vi "Desktop Main.vi"() -> ()   [LabVIEW 2019]
doc: "Sends commands and instructions through UDP communication to the myRIO in order to move the motors"
panel:
  out "Tab of colors":i32[][](array[numeric])
  out "Camera 4":T1(plugin-control)
  out "Camera 3":T1(plugin-control)
  out "Camera 2":T1(plugin-control)
  out "Camera 1":T1(plugin-control)
  in  "RESET":bool
  out "Random":string[](array[string])
  out "Commands to Execute":string[](array[string])
  out "Time to execute \n(in second)":dbl(slide) scale=0.014..14.0
  in  "Speed":string(combo)="Slow"
  in  "Difficulty for random":string(combo)="Easy"
  in  "Unrandomize":bool
  in  "Random":bool
  in  "Touche U'":bool
  in  "Touche U":bool
  in  "Touche D'":bool
  in  "Touche D":bool
  in  "Touche L'":bool
  in  "Touche L":bool
  in  "Touche B'":bool
  in  "Touche B":bool
  in  "Touche R'":bool
  in  "Touche F'":bool
  in  "Touche R":bool
  in  "Solve":bool
  in  "Touche F":bool
  in  "Tab cmd forcées":string[](array[string])
  in  "GO Tableau forcé":bool
  in  "Stop Button":bool
  out "error out":errorcluster
  in  "Target IP Address":string="172.22.11.2"
  # "Overview: Resolve a Rubik's cube or send some commands using User Datagram Protocol (UDP). The data of this \"Desktop Main\" is sent to the myRIO target.\n\nInstructions:\n1. Ensure RT Main.vi is already running.\n2. Run this VI.\n3. Click on the function you want.\n4. Observe the Rubik's cube moving.\n5. Click Stop to stop both VIs."
  # "Move a face"
  # "Difficulty for randomize"
  # "Easy : 5 moves\nMedium : 15 moves\nHard : 25 moves\nHardcore : 50 moves"
  # "List of commands to execute"
  # "1. Write in the tab the commands you want to execute\n    (F, F', L, L', R, R', B, B', U, U', D, D')\n\n2. Click on \"LAUNCH\"\n\n3. Click on \"RESET COMMANDS\" to reset the keys you entered"
  # "s"
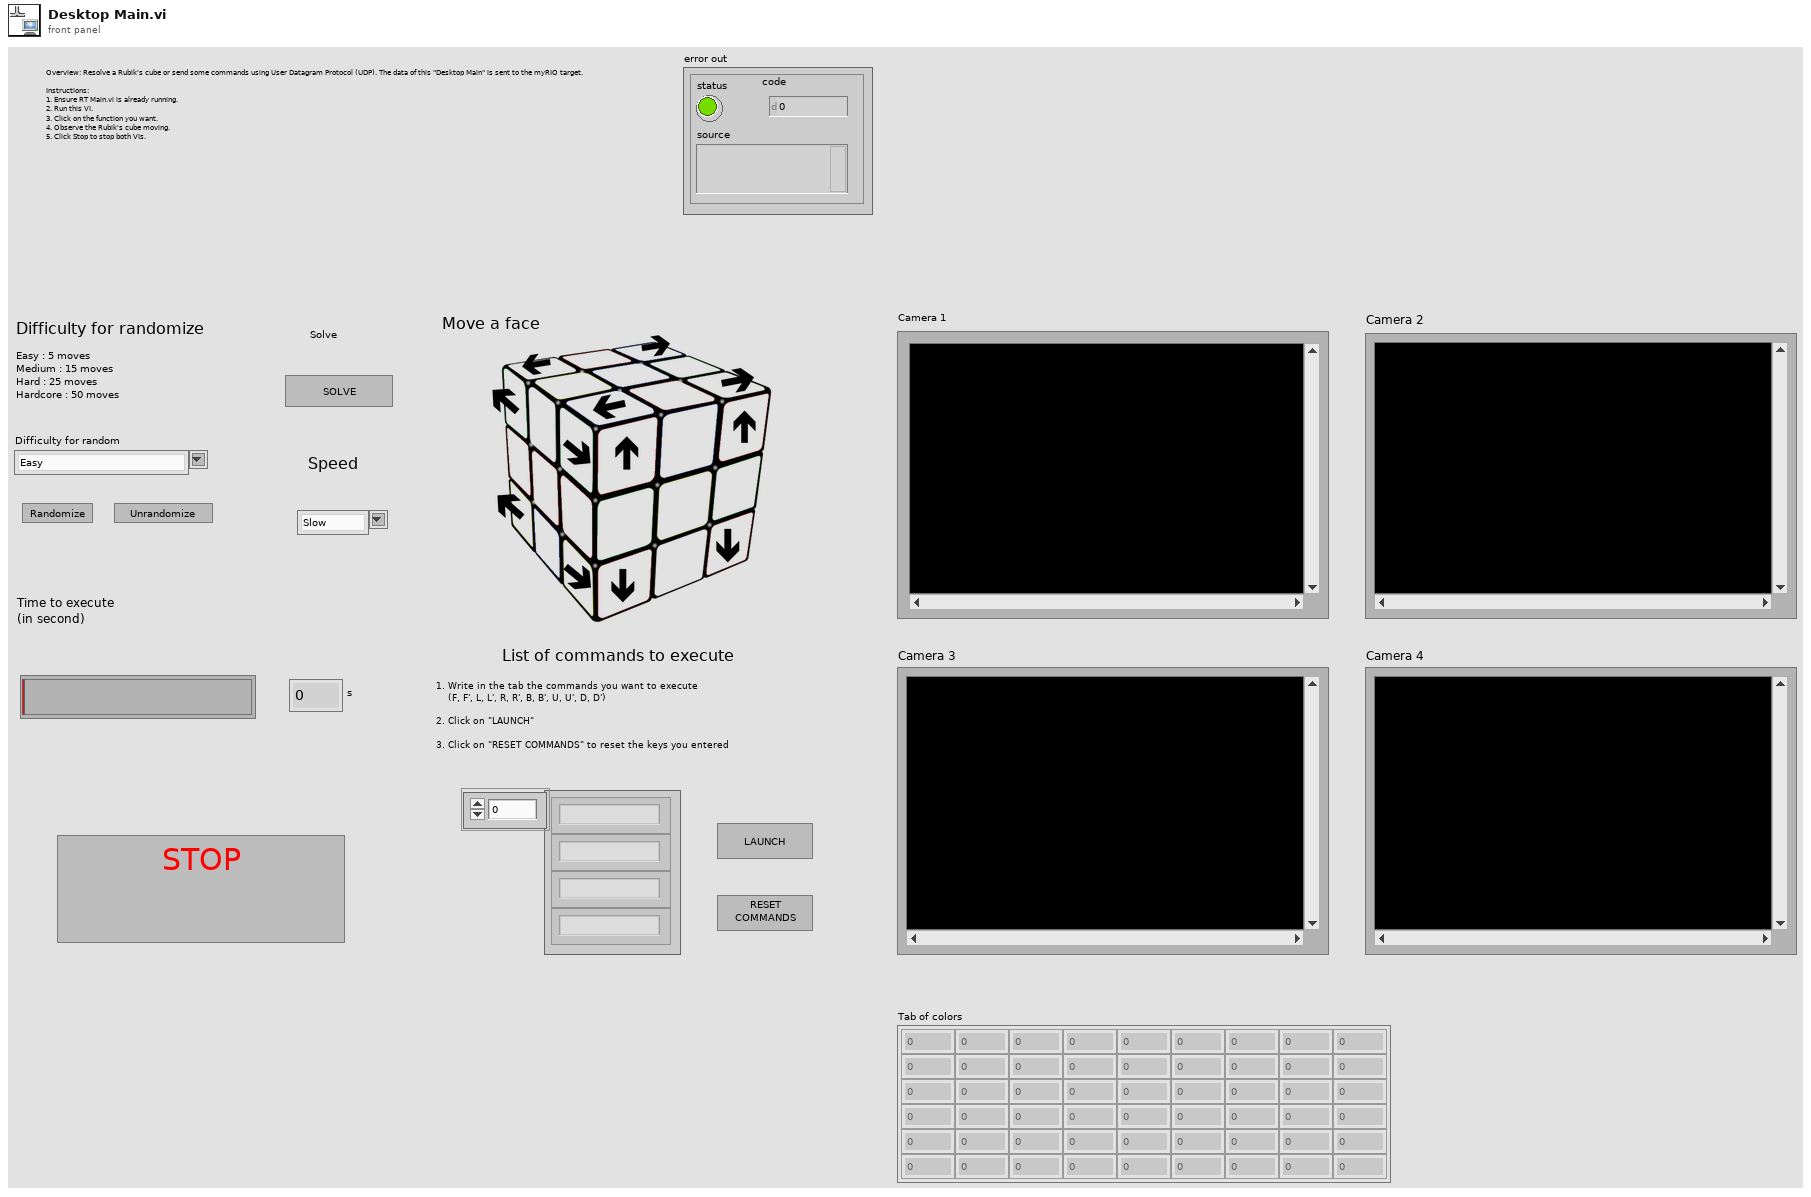
[diagram p1: front panel]
types:
  T1 = typedef "IMAQ Image.ctl" = refnum<image>
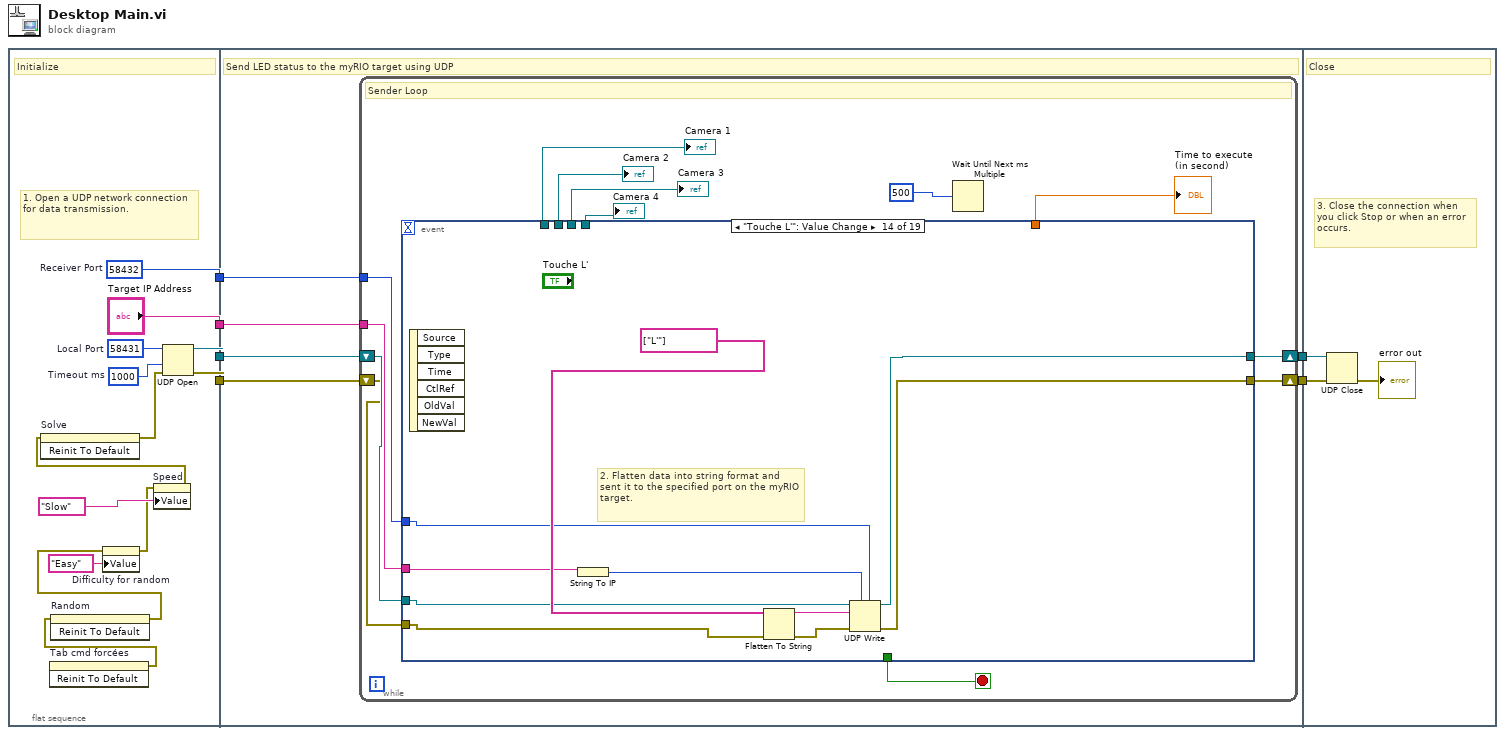
[diagram p0: block diagram]
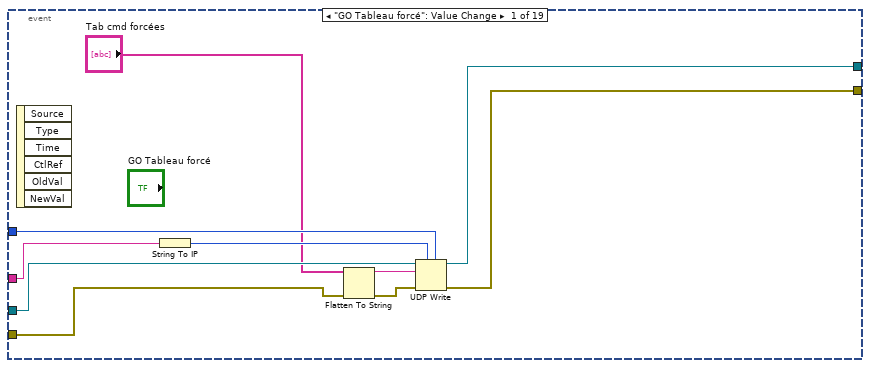
[diagram p2: hidden frame]
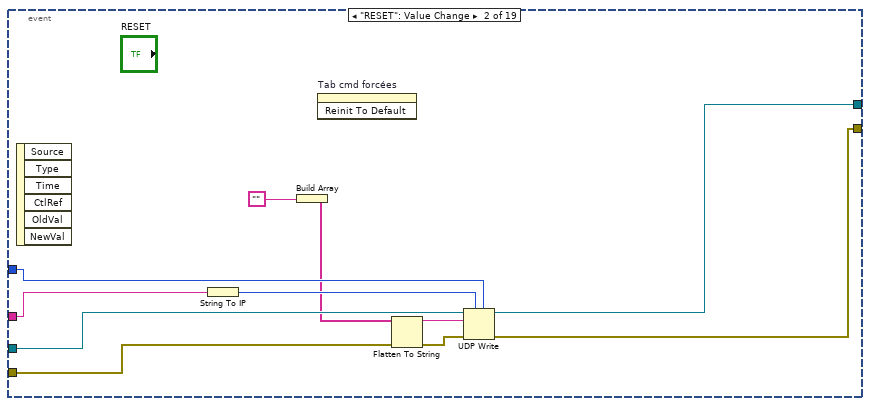
[diagram p3: hidden frame]
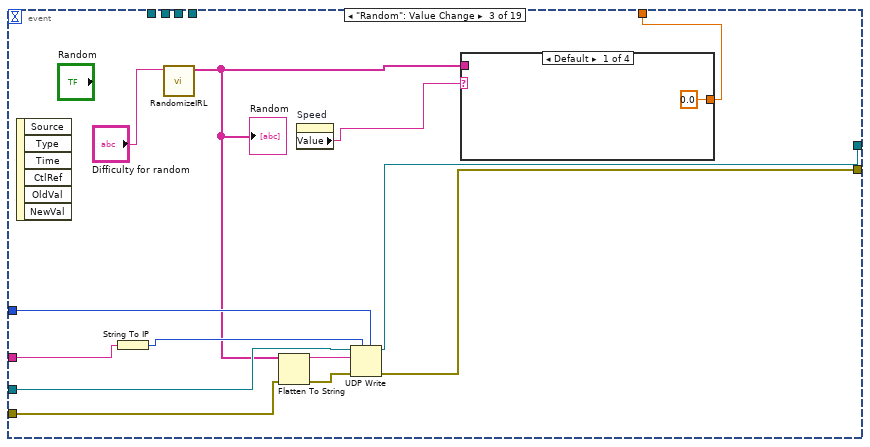
[diagram p4: hidden frame]
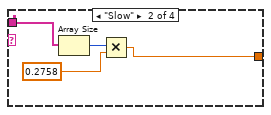
[diagram p5: hidden frame]
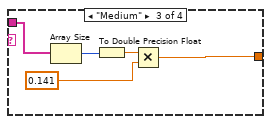
[diagram p6: hidden frame]
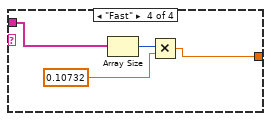
[diagram p7: hidden frame]
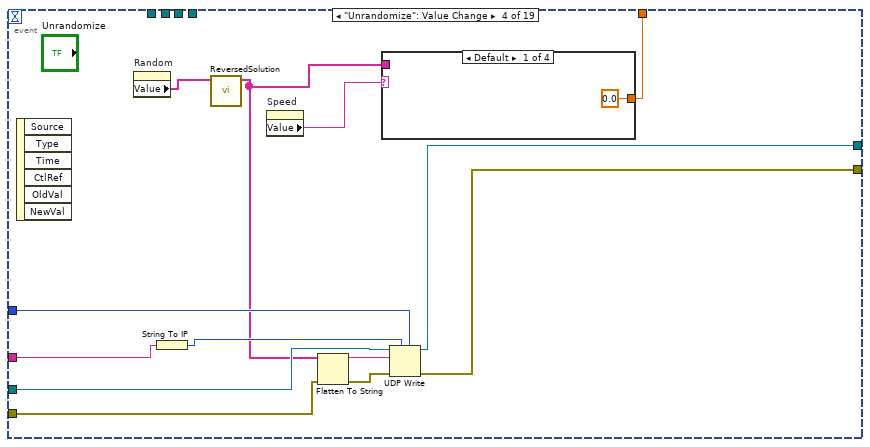
[diagram p8: hidden frame]
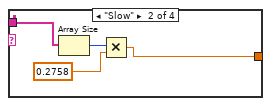
[diagram p9: hidden frame]
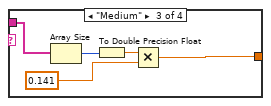
[diagram p10: hidden frame]
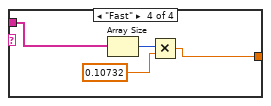
[diagram p11: hidden frame]
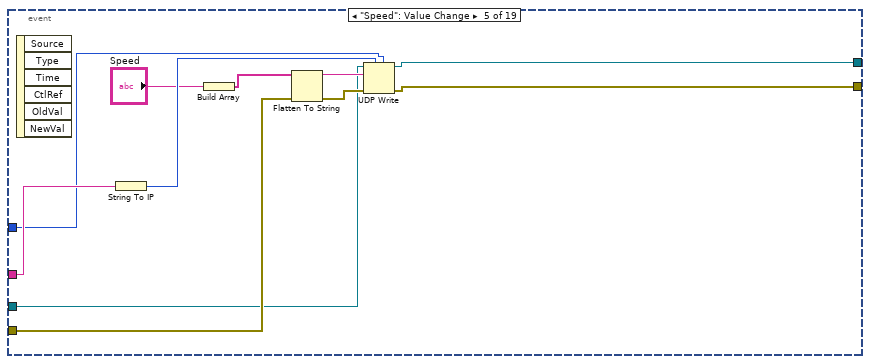
[diagram p12: hidden frame]
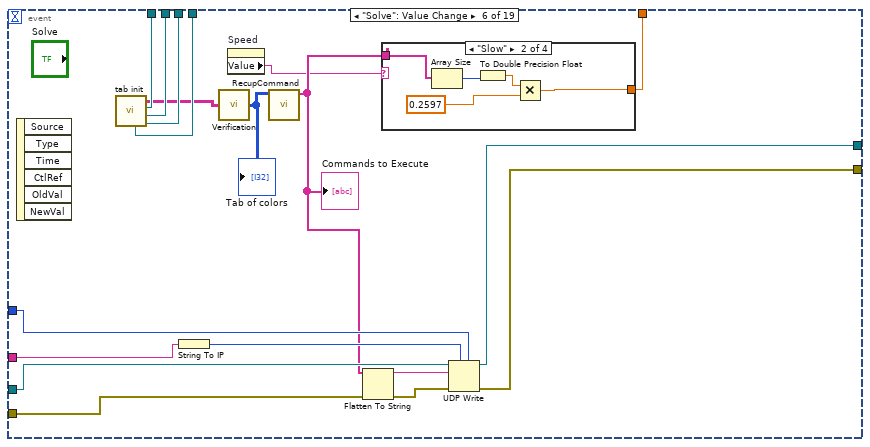
[diagram p13: hidden frame]
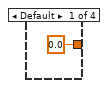
[diagram p14: hidden frame]
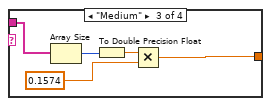
[diagram p15: hidden frame]
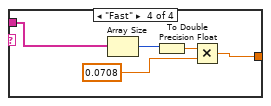
[diagram p16: hidden frame]
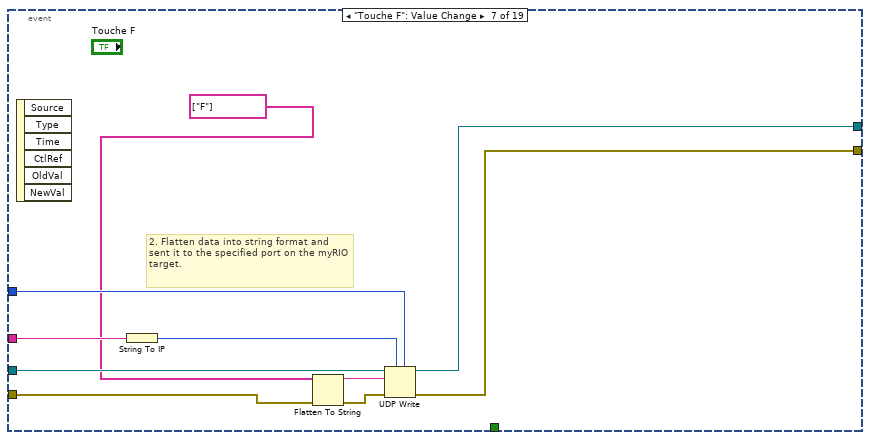
[diagram p17: hidden frame]
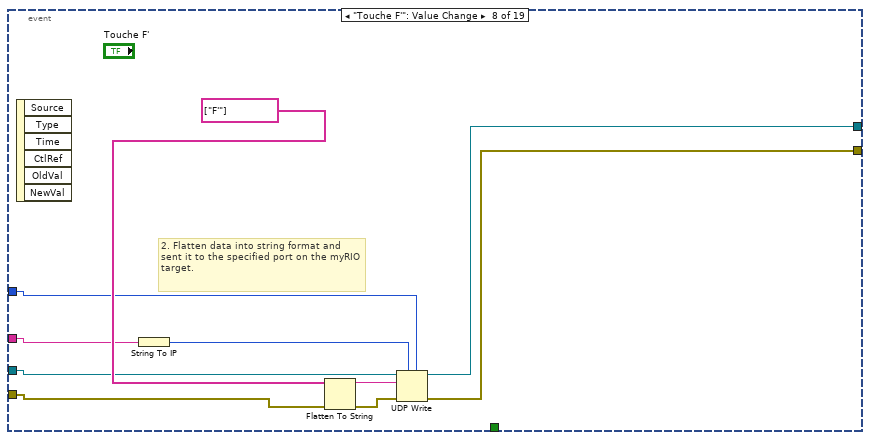
[diagram p18: hidden frame]
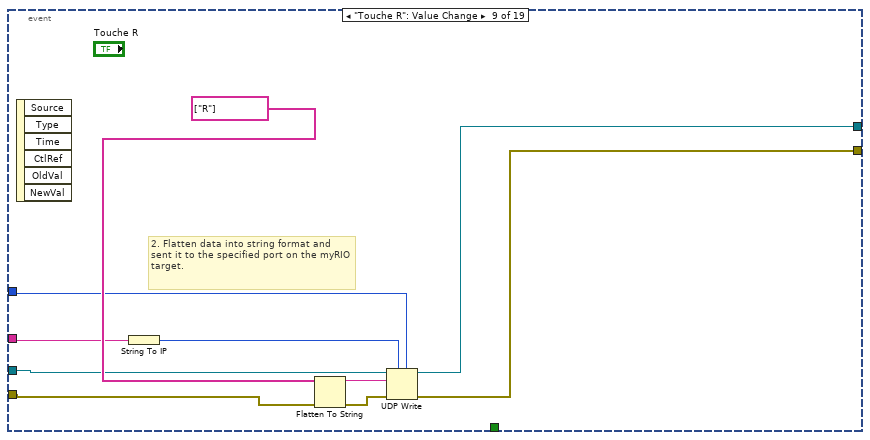
[diagram p19: hidden frame]
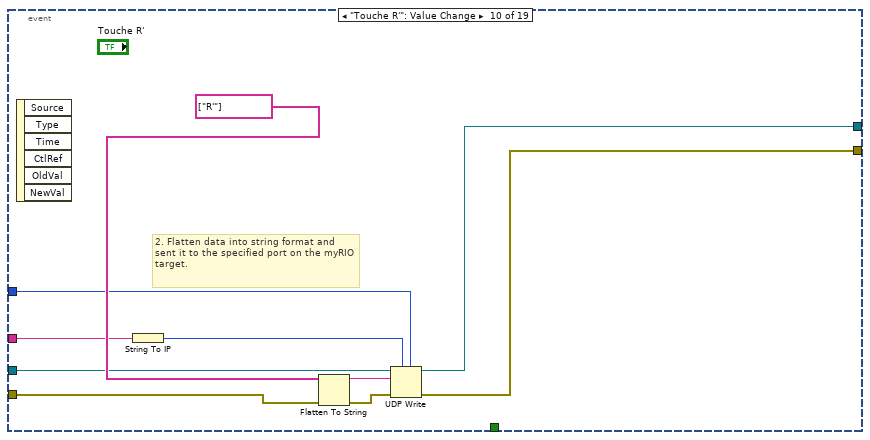
[diagram p20: hidden frame]
diagram:
  n1 = flat-sequence {
    tunnel: [w18] -> w4
    tunnel: [w17] -> w3
    tunnel: ["Target IP Address"] -> w2
    tunnel: [w15] -> w1
    tunnel: [w25] -> w6
    tunnel: [w24] -> w5
    tunnel: w4 -> [w23]
    tunnel: w3 -> [w22]
    tunnel: w2 -> [w21]
    tunnel: w1 -> [w20]
    tunnel: w6 -> [w291]
    tunnel: w5 -> [w292]
    frame #0 {
      w14 = 1000  # Timeout ms
      w15 = u16 58432  # Receiver Port
      w19 = u16 58431  # Local Port
      # "1. Open a UDP network connection for data transmission."
      # "Initialize"
      n2 = invoke on="Tab cmd forcées" class="Arr (strict)" method="Reinit To Default"() -> (error out=w7:errorcluster)  [unwired: 3 in, 2 out]
      n3 = invoke on="Random" class="Arr (strict)" method="Reinit To Default"(error in=w7) -> (error out=w8:errorcluster)  [unwired: 2 in, 2 out]
      n4 = property on="Difficulty for random" class="CmbBox"(error in=w8, "Value"="Easy" ("Difficulty for random")) -> (error out=w10:errorcluster)  [unwired: 1 in, 1 out]
      n5 = property on="Speed" class="CmbBox"(error in=w10, "Value"="Slow" ("Speed")) -> (error out=w9:errorcluster)  [unwired: 1 in, 1 out]
      n6 = invoke on="Solve" class="Bool" method="Reinit To Default"(error in=w9) -> (error out=w13:errorcluster)  [unwired: 2 in, 2 out]
      n7 = UDP Open(8:w13, 9:w14, 11:w19) -> (port=w18:refnum<k16>, 0:w17:errorcluster)  [unwired: 2 in, 1 out]
    }
    frame #1 {
      # "Send LED status to the myRIO target using UDP"
      n8 = while {
        shift-right: [w37] -> w25
        shift-left: w22 -> [w32]
        shift-right: [w36] -> w24
        shift-left: w23 -> [w33]
        tunnel: w21 -> [w34]
        tunnel: w20 -> [w35]
        stop <- w31 stop-if-true
        # "Sender Loop"
        n9 = event shown="[13] \"Touche L'\": Value Change" {
          selector: _ -> [_ _ _ _ _ _ _ _ _ _ _ _ _ _ _ _ _ _ _]
          dyn-events: _ -> [_ _ _ _ _ _ _ _ _ _ _ _ _ _ _ _ _ _ _]
          timeout: _ -> [_ _ _ _ _ _ _ _ _ _ _ _ _ _ _ _ _ _ _]
          tunnel: [w39 w52 w64 w91 w119 w135 w165 w169 w180 w193 w203 w213 w221 w229 w240 w253 w263 w273 w284] -> w37
          tunnel: [w40 w51 w65 w92 w118 w134 w164 w174 w179 w194 w204 w214 w222 w230 w241 w254 w264 w274 w285] -> w36
          tunnel: w35 -> [w44 w56 w66 w93 w116 w138 w163 w173 w184 w189 w202 w212 w224 w234 w239 w252 w262 w272 w280]
          tunnel: w34 -> [w45 w55 w70 w94 w122 w139 w162 w172 w183 w190 w201 w211 w223 w233 w244 w251 w261 w271 w282]
          tunnel: w33 -> [w43 w54 w68 w95 w117 w137 w161 w171 w182 w191 w200 w210 w219 w232 w243 w250 w260 w270 w279]
          tunnel: w32 -> [w42 w53 w67 w96 w120 w136 w160 w170 w181 w192 w199 w209 w220 w231 w242 w249 w259 w269 w281]
          tunnel: [_ _ _ _ _ _ _ _ _ _ _ _ _ _ _ _ _ _ "Stop Button"] -> w31
          tunnel: [_ _ w62 w89 _ w131 _ _ _ _ _ _ _ _ _ _ _ _ _] -> w26
          tunnel: [_ _ _ _ _ w130 _ _ _ _ _ _ _ _ _ _ _ _ _] -> w30
          tunnel: [_ _ _ _ _ w129 _ _ _ _ _ _ _ _ _ _ _ _ _] -> w29
          tunnel: [_ _ _ _ _ w128 _ _ _ _ _ _ _ _ _ _ _ _ _] -> w27
          tunnel: [_ _ _ _ _ w127 _ _ _ _ _ _ _ _ _ _ _ _ _] -> w28
          event "GO Tableau forcé": Value Change {
            n10 = event-data() -> ()  [unwired: 1 in, 6 out]
            n11 = String To IP(1:w45) -> (0:w48:u32)
            n12 = Flatten To String(anything="Tab cmd forcées", error in (no error)=w42) -> (data string=w47:string, error out=w46:errorcluster)  [unwired: 2 in, 1 out]
            n13 = UDP Write(address=w48, port or service name=w44, connection ID=w43, data in=w47, 8:w46) -> (error out=w39:errorcluster, 3:w40:refnum<k16>)  [unwired: 1 in]
          }
          event "RESET": Value Change {
            n14 = event-data() -> ()  [unwired: 1 in, 6 out]
            n15 = String To IP(1:w55) -> (0:w59:u32)
            n16 = Build Array("") -> (w49:string[])
            n17 = invoke on="Tab cmd forcées" class="Arr (strict)" method="Reinit To Default"() -> ()  [unwired: 3 in, 3 out]
            n18 = Flatten To String(anything=w49, error in (no error)=w53) -> (data string=w58:string, error out=w57:errorcluster)  [unwired: 2 in, 1 out]
            n19 = UDP Write(address=w59, port or service name=w56, connection ID=w54, data in=w58, 8:w57) -> (error out=w52:errorcluster, 3:w51:refnum<k16>)  [unwired: 1 in]
          }
          event "Random": Value Change {
            n20 = event-data() -> ()  [unwired: 1 in, 6 out]
            n21 = String To IP(1:w70) -> (0:w69:u32)
            n22 = call "RandomizeIRL.vi"("Difficulty"="Difficulty for random") -> ("appended array 2"=w61:string[])  [unwired: 10 in]
            "Random" <- w61
            n23 = Flatten To String(anything=w61, error in (no error)=w67) -> (data string=w72:string, error out=w71:errorcluster)  [unwired: 2 in, 1 out]
            n24 = property on="Speed" class="CmbBox"() -> ("Value"=w60:string)  [unwired: 2 in, 2 out]
            n25 = UDP Write(address=w69, port or service name=w66, connection ID=w68, data in=w72, 8:w71) -> (error out=w64:errorcluster, 3:w65:refnum<k16>)  [unwired: 1 in]
            n26 = case shown="Default" w60 {
              tunnel: [0.0 w77 w82 w86] -> w62
              tunnel: w61 -> [_ w76 w81 w85]
              frame Default {
              }
              frame "Slow" {
                n27 = Array Size(array=w76) -> (size(s)=w74:i32)
                n28 = Multiply(x=w74, y=0.2758) -> (x*y=w77:dbl)
              }
              frame "Medium" {
                n29 = Array Size(array=w81) -> (size(s)=w78:i32)
                n30 = To Double Precision Float(number=w78) -> (double precision float=w80:dbl)
                n31 = Multiply(x=w80, y=0.141) -> (x*y=w82:dbl)
              }
              frame "Fast" {
                n32 = Array Size(array=w85) -> (size(s)=w83:i32)
                n33 = Multiply(x=w83, y=0.10732) -> (x*y=w86:dbl)
              }
            }
          }
          event "Unrandomize": Value Change {
            n34 = event-data() -> ()  [unwired: 1 in, 6 out]
            n35 = property on="Random" class="Arr (strict)"() -> ("Value"=w90:string[])  [unwired: 2 in, 2 out]
            n36 = String To IP(1:w94) -> (0:w97:u32)
            n37 = call "ReversedSolution.vi"("Array"=w90) -> ("Array 2"=w88:string[])  [unwired: 10 in]
            n38 = property on="Speed" class="CmbBox"() -> ("Value"=w87:string)  [unwired: 2 in, 2 out]
            n39 = Flatten To String(anything=w88, error in (no error)=w96) -> (data string=w99:string, error out=w98:errorcluster)  [unwired: 2 in, 1 out]
            n40 = case shown="Default" w87 {
              tunnel: [0.0 w103 w108 w112] -> w89
              tunnel: w88 -> [_ w102 w107 w111]
              frame Default {
              }
              frame "Slow" {
                n41 = Array Size(array=w102) -> (size(s)=w101:i32)
                n42 = Multiply(x=w101, y=0.2758) -> (x*y=w103:dbl)
              }
              frame "Medium" {
                n43 = Array Size(array=w107) -> (size(s)=w105:i32)
                n44 = To Double Precision Float(number=w105) -> (double precision float=w106:dbl)
                n45 = Multiply(x=w106, y=0.141) -> (x*y=w108:dbl)
              }
              frame "Fast" {
                n46 = Array Size(array=w111) -> (size(s)=w110:i32)
                n47 = Multiply(x=w110, y=0.10732) -> (x*y=w112:dbl)
              }
            }
            n48 = UDP Write(address=w97, port or service name=w93, connection ID=w95, data in=w99, 8:w98) -> (error out=w91:errorcluster, 3:w92:refnum<k16>)  [unwired: 1 in]
          }
          event "Speed": Value Change {
            n49 = event-data() -> ()  [unwired: 1 in, 6 out]
            n50 = String To IP(1:w122) -> (0:w121:u32)
            n51 = Build Array("Speed") -> (w115:string[])
            n52 = Flatten To String(anything=w115, error in (no error)=w120) -> (data string=w124:string, error out=w123:errorcluster)  [unwired: 2 in, 1 out]
            n53 = UDP Write(address=w121, port or service name=w116, connection ID=w117, data in=w124, 8:w123) -> (error out=w119:errorcluster, 3:w118:refnum<k16>)  [unwired: 1 in]
          }
          event "Solve": Value Change {
            n54 = event-data() -> ()  [unwired: 1 in, 6 out]
            n55 = call "tab init.vi"() -> ("Image 3"=w128:T1, "Image 2"=w129:T1, "Image"=w130:T1, "appended array"=w126:string[][], "Image 4"=w127:T1)  [unwired: 7 in]
            n56 = String To IP(1:w139) -> (0:w142:u32)
            n57 = call "Verification.vi"("appended array 2"=w126) -> ("Array"=w125:i32[][])
            "Tab of colors" <- w125
            n58 = property on="Speed" class="CmbBox"() -> ("Value"=w132:string)  [unwired: 2 in, 2 out]
            n59 = call "RecupCommand.vi"("Rubix initialisé via caméra"=w125) -> ("Commands to Execute"=w133:string[])  [unwired: 10 in]
            "Commands to Execute" <- w133
            n60 = Flatten To String(anything=w133, error in (no error)=w136) -> (data string=w141:string, error out=w140:errorcluster)  [unwired: 2 in, 1 out]
            n61 = case shown="\"Slow\"" w132 {
              tunnel: [0.0 w147 w152 w157] -> w131
              tunnel: w133 -> [_ w146 w151 w156]
              frame Default {
              }
              frame "Slow" {
                n62 = Array Size(array=w146) -> (size(s)=w144:i32)
                n63 = To Double Precision Float(number=w144) -> (double precision float=w145:dbl)
                n64 = Multiply(x=w145, y=0.2597) -> (x*y=w147:dbl)
              }
              frame "Medium" {
                n65 = Array Size(array=w151) -> (size(s)=w149:i32)
                n66 = To Double Precision Float(number=w149) -> (double precision float=w150:dbl)
                n67 = Multiply(x=w150, y=0.1574) -> (x*y=w152:dbl)
              }
              frame "Fast" {
                n68 = Array Size(array=w156) -> (size(s)=w154:i32)
                n69 = To Double Precision Float(number=w154) -> (double precision float=w155:dbl)
                n70 = Multiply(x=w155, y=0.0708) -> (x*y=w157:dbl)
              }
            }
            n71 = UDP Write(address=w142, port or service name=w138, connection ID=w137, data in=w141, 8:w140) -> (error out=w135:errorcluster, 3:w134:refnum<k16>)  [unwired: 1 in]
          }
          event "Touche F": Value Change {
            # "2. Flatten data into string format and\nsent it to the specified port on the myRIO target."
            n72 = event-data() -> ()  [unwired: 1 in, 6 out]
            n73 = String To IP(1:w162) -> (0:w168:u32)
            n74 = Flatten To String(anything=string[] ["F"], error in (no error)=w160) -> (data string=w167:string, error out=w166:errorcluster)  [unwired: 2 in, 1 out]
            n75 = UDP Write(address=w168, port or service name=w163, connection ID=w161, data in=w167, 8:w166) -> (error out=w165:errorcluster, 3:w164:refnum<k16>)  [unwired: 1 in]
          }
          event "Touche F'": Value Change {
            # "2. Flatten data into string format and\nsent it to the specified port on the myRIO target."
            n76 = event-data() -> ()  [unwired: 1 in, 6 out]
            n77 = String To IP(1:w172) -> (0:w178:u32)
            n78 = Flatten To String(anything=string[] ["F'"], error in (no error)=w170) -> (data string=w177:string, error out=w176:errorcluster)  [unwired: 2 in, 1 out]
            n79 = UDP Write(address=w178, port or service name=w173, connection ID=w171, data in=w177, 8:w176) -> (error out=w169:errorcluster, 3:w174:refnum<k16>)  [unwired: 1 in]
          }
          event "Touche R": Value Change {
            # "2. Flatten data into string format and\nsent it to the specified port on the myRIO target."
            n80 = event-data() -> ()  [unwired: 1 in, 6 out]
            n81 = String To IP(1:w183) -> (0:w188:u32)
            n82 = Flatten To String(anything=string[] ["R"], error in (no error)=w181) -> (data string=w187:string, error out=w186:errorcluster)  [unwired: 2 in, 1 out]
            n83 = UDP Write(address=w188, port or service name=w184, connection ID=w182, data in=w187, 8:w186) -> (error out=w180:errorcluster, 3:w179:refnum<k16>)  [unwired: 1 in]
          }
          event "Touche R'": Value Change {
            # "2. Flatten data into string format and\nsent it to the specified port on the myRIO target."
            n84 = event-data() -> ()  [unwired: 1 in, 6 out]
            n85 = String To IP(1:w190) -> (0:w198:u32)
            n86 = Flatten To String(anything=string[] ["R'"], error in (no error)=w192) -> (data string=w197:string, error out=w196:errorcluster)  [unwired: 2 in, 1 out]
            n87 = UDP Write(address=w198, port or service name=w189, connection ID=w191, data in=w197, 8:w196) -> (error out=w193:errorcluster, 3:w194:refnum<k16>)  [unwired: 1 in]
          }
          event "Touche B": Value Change {
            # "2. Flatten data into string format and\nsent it to the specified port on the myRIO target."
            n88 = event-data() -> ()  [unwired: 1 in, 6 out]
            n89 = String To IP(1:w201) -> (0:w208:u32)
            n90 = Flatten To String(anything=string[] ["B"], error in (no error)=w199) -> (data string=w207:string, error out=w206:errorcluster)  [unwired: 2 in, 1 out]
            n91 = UDP Write(address=w208, port or service name=w202, connection ID=w200, data in=w207, 8:w206) -> (error out=w203:errorcluster, 3:w204:refnum<k16>)  [unwired: 1 in]
          }
          event "Touche B'": Value Change {
            # "2. Flatten data into string format and\nsent it to the specified port on the myRIO target."
            n92 = event-data() -> ()  [unwired: 1 in, 6 out]
            n93 = String To IP(1:w211) -> (0:w218:u32)
            n94 = Flatten To String(anything=string[] ["B'"], error in (no error)=w209) -> (data string=w217:string, error out=w216:errorcluster)  [unwired: 2 in, 1 out]
            n95 = UDP Write(address=w218, port or service name=w212, connection ID=w210, data in=w217, 8:w216) -> (error out=w213:errorcluster, 3:w214:refnum<k16>)  [unwired: 1 in]
          }
          event "Touche L": Value Change {
            # "2. Flatten data into string format and\nsent it to the specified port on the myRIO target."
            n96 = event-data() -> ()  [unwired: 1 in, 6 out]
            n97 = String To IP(1:w223) -> (0:w228:u32)
            n98 = Flatten To String(anything=string[] ["L"], error in (no error)=w220) -> (data string=w227:string, error out=w226:errorcluster)  [unwired: 2 in, 1 out]
            n99 = UDP Write(address=w228, port or service name=w224, connection ID=w219, data in=w227, 8:w226) -> (error out=w221:errorcluster, 3:w222:refnum<k16>)  [unwired: 1 in]
          }
          event "Touche L'": Value Change {
            # "2. Flatten data into string format and\nsent it to the specified port on the myRIO target."
            n100 = event-data() -> ()  [unwired: 1 in, 6 out]
            n101 = String To IP(1:w233) -> (0:w238:u32)
            n102 = Flatten To String(anything=string[] ["L'"], error in (no error)=w231) -> (data string=w237:string, error out=w236:errorcluster)  [unwired: 2 in, 1 out]
            n103 = UDP Write(address=w238, port or service name=w234, connection ID=w232, data in=w237, 8:w236) -> (error out=w229:errorcluster, 3:w230:refnum<k16>)  [unwired: 1 in]
          }
          event "Touche D": Value Change {
            # "2. Flatten data into string format and\nsent it to the specified port on the myRIO target."
            n104 = event-data() -> ()  [unwired: 1 in, 6 out]
            n105 = String To IP(1:w244) -> (0:w248:u32)
            n106 = Flatten To String(anything=string[] ["D"], error in (no error)=w242) -> (data string=w247:string, error out=w246:errorcluster)  [unwired: 2 in, 1 out]
            n107 = UDP Write(address=w248, port or service name=w239, connection ID=w243, data in=w247, 8:w246) -> (error out=w240:errorcluster, 3:w241:refnum<k16>)  [unwired: 1 in]
          }
          event "Touche D'": Value Change {
            # "2. Flatten data into string format and\nsent it to the specified port on the myRIO target."
            n108 = event-data() -> ()  [unwired: 1 in, 6 out]
            n109 = String To IP(1:w251) -> (0:w258:u32)
            n110 = Flatten To String(anything=string[] ["D'"], error in (no error)=w249) -> (data string=w257:string, error out=w256:errorcluster)  [unwired: 2 in, 1 out]
            n111 = UDP Write(address=w258, port or service name=w252, connection ID=w250, data in=w257, 8:w256) -> (error out=w253:errorcluster, 3:w254:refnum<k16>)  [unwired: 1 in]
          }
          event "Touche U": Value Change {
            # "2. Flatten data into string format and\nsent it to the specified port on the myRIO target."
            n112 = event-data() -> ()  [unwired: 1 in, 6 out]
            n113 = String To IP(1:w261) -> (0:w268:u32)
            n114 = Flatten To String(anything=string[] ["U"], error in (no error)=w259) -> (data string=w267:string, error out=w266:errorcluster)  [unwired: 2 in, 1 out]
            n115 = UDP Write(address=w268, port or service name=w262, connection ID=w260, data in=w267, 8:w266) -> (error out=w263:errorcluster, 3:w264:refnum<k16>)  [unwired: 1 in]
          }
          event "Touche U'": Value Change {
            # "2. Flatten data into string format and\nsent it to the specified port on the myRIO target."
            n116 = event-data() -> ()  [unwired: 1 in, 6 out]
            n117 = String To IP(1:w271) -> (0:w278:u32)
            n118 = Flatten To String(anything=string[] ["U'"], error in (no error)=w269) -> (data string=w277:string, error out=w276:errorcluster)  [unwired: 2 in, 1 out]
            n119 = UDP Write(address=w278, port or service name=w272, connection ID=w270, data in=w277, 8:w276) -> (error out=w273:errorcluster, 3:w274:refnum<k16>)  [unwired: 1 in]
          }
          event "Stop Button": Value Change {
            # "2. Flatten data into string format and\nsent it to the specified port on the myRIO target."
            n120 = event-data() -> ()  [unwired: 1 in, 6 out]
            n121 = String To IP(1:w282) -> (0:w288:u32)
            n122 = Flatten To String(anything=string[] ["STOP"], error in (no error)=w281) -> (data string=w287:string, error out=w286:errorcluster)  [unwired: 2 in, 1 out]
            n123 = UDP Write(address=w288, port or service name=w280, connection ID=w279, data in=w287, 8:w286) -> (error out=w284:errorcluster, 3:w285:refnum<k16>)  [unwired: 1 in]
          }
        }
        "Time to execute \n(in second)" <- w26
        "Camera 1" <- w30
        "Camera 2" <- w29
        "Camera 3" <- w27
        "Camera 4" <- w28
        n124 = Wait Until Next ms Multiple(millisecond multiple=u32 500) -> ()  [unwired: 1 out]
      }
    }
    frame #2 {
      # "3. Close the connection when you click Stop or when an error occurs."
      # "Close"
      n125 = UDP Close(connection ID=w292, 8:w291) -> (error out=→"error out":errorcluster)  [unwired: 1 out]
    }
  }
